vi "FRIC_navX_Get_HaultStatus.vi"(7 "Update":bool) -> (3 "Hault":bool)   [LabVIEW 2015]
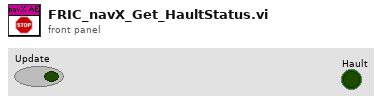
[diagram p1: front panel]
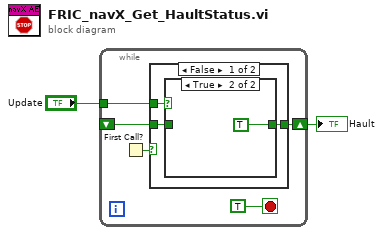
[diagram p0: block diagram]
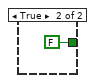
[diagram p3: hidden frame]
diagram:
  n1 = while {
    shift-right: [w7] -> w1
    shift-left: _ -> [w5]
    tunnel: "Update" -> [w6]
    stop <- TRUE stop-if-true
    n2 = First Call?() -> (First Call?: T/F=w3:bool)
    n3 = case shown="False" w3 {
      tunnel: [w10 FALSE] -> w7
      tunnel: w6 -> [w9 _]
      tunnel: w5 -> [w8 _]
      frame False {
        n4 = case shown="True" w9 {
          tunnel: [w11 TRUE] -> w10
          tunnel: w8 -> [w11 _]
          frame False {
          }
          frame True {
          }
        }
      }
      frame True {
      }
    }
  }
  "Hault" <- w1
